vi "check if running.vi"(8 "error in (no error)":errorcluster, 11 "CL57RS in":refnum<class "CL57RS.lvclass">) -> (0 "error out":errorcluster, 2 "Running?":bool, 3 "CL57RS out":refnum<class "CL57RS.lvclass">)   [LabVIEW 2025, in "Motor.lvlib" / "CL57RS.lvclass"]
uses:
  CL57RS.lvclass
  CL57RS.lvclass/CL57RS.ctl
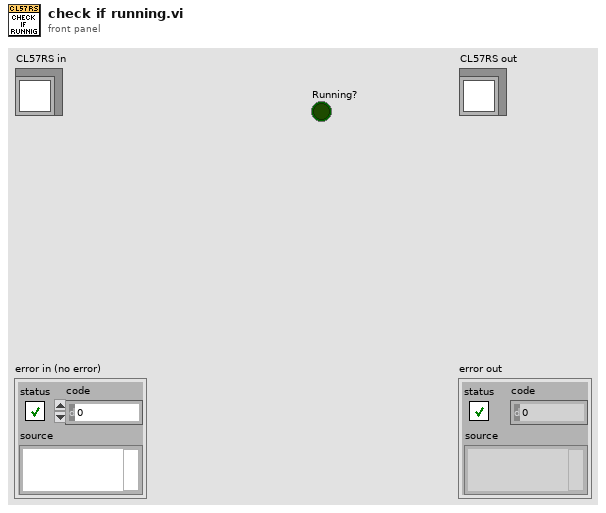
[diagram p1: front panel]
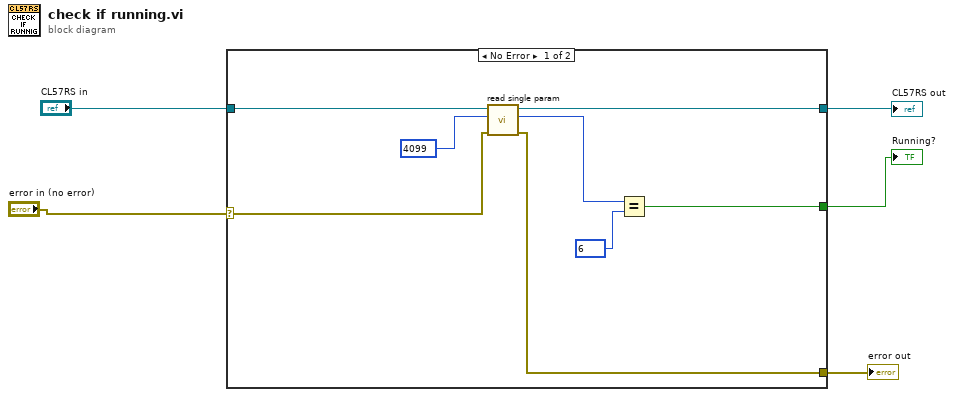
[diagram p0: block diagram]
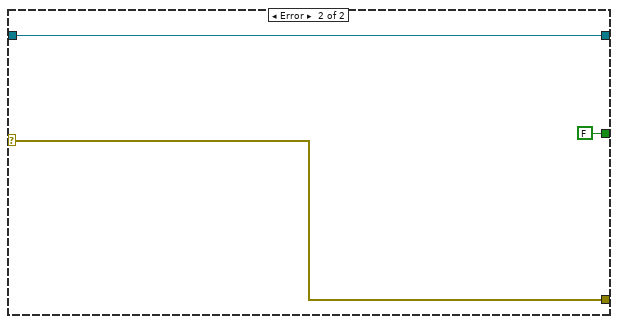
[diagram p2: hidden frame]
diagram:
  n1 = case shown="No Error" "error in (no error)" {
    selector: "error in (no error)" -> [w8 w16]
    tunnel: [w7 w16] -> w1
    tunnel: [w10 w15] -> w5
    tunnel: "CL57RS in" -> [w11 w15]
    tunnel: [w12 FALSE] -> w2
    frame No Error {
      n2 = call "read single param.vi"("error in (no error)"=w8, "address"=u16 4099, "CL57RS in"=w11) -> ("error out"=w7:errorcluster, "register"=w6:u16, "CL57RS out"=w10:refnum<class "CL57RS.lvclass">)  [unwired: 6 in]
      n3 = Equal?(x=w6, y=u16 6 ("address")) -> (x = y?=w12:bool)
    }
    frame Error {
    }
  }
  "error out" <- w1
  "CL57RS out" <- w5
  "Running?" <- w2
